vi "Async Start VI by Ref.vi"(8 "GUI.lvlib:GUI.lvclass":refnum<class "GUI.lvclass">, 11 "Static VI reference":refnum<vi>) -> ()   [LabVIEW 2020, in "GUI.lvlib" / "GUI.lvclass"]
uses:
  GUI.lvclass
panel:
  out "error out":errorcluster
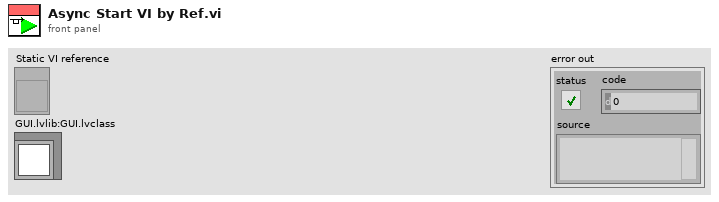
[diagram p1: front panel]
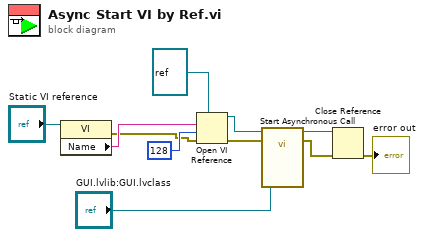
[diagram p0: block diagram]
diagram:
  n1 = property class="VI"(reference="Static VI reference") -> (error out=w5:errorcluster, "Name"=w7:string)  [unwired: 1 in, 1 out]
  n2 = Open VI Reference(type specifier VI Refnum (for type only)=refnum<vi> refnum, vi path=w7, options=128, error in (no error)=w5) -> (vi reference=w11:refnum<vi>, error out=w4:errorcluster)  [unwired: 2 in]
  n3 = call-by-ref "Start Asynchronous Call"(reference=w11, error in=w4, "GUI.lvlib:GUI.lvclass"="GUI.lvlib:GUI.lvclass") -> (reference out=w8:refnum<vi>, error out=w3:errorcluster)  [unwired: 11 in]
  n4 = Close Reference(reference=w8, error in (no error)=w3) -> (error out=→"error out":errorcluster)
